vi "抽取1D数组(CTRL-REF).vi"(8 "error in (no error)":errorcluster caption="错误输入（无错误）", 10 "n":i32, 11 "输入数组":refnum<vi>[](array[refnum])) -> (0 "error out":errorcluster caption="错误输出", 3 "输出数组":refnum<vi>[][](array[refnum]))   [LabVIEW 2012]
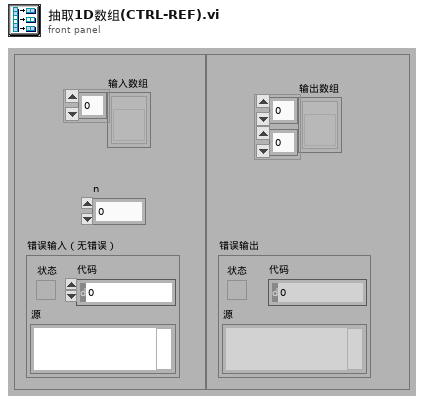
[diagram p1: front panel]
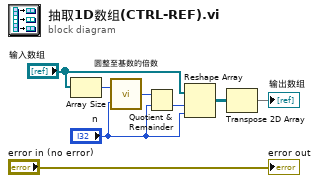
[diagram p0: block diagram]
diagram:
  n1 = Array Size(array="输入数组") -> (size(s)=w7:i32)
  n2 = call "圆整至基数的倍数.vi"("base"="n", "input"=w7) -> ("output"=w3:i32)
  n3 = Quotient & Remainder(x=w3, y="n") -> (floor(x/y)=w1:i32)  [unwired: 1 out]
  n4 = Reshape Array("输入数组", w1, "n") -> (w6:refnum<vi>[][])
  n5 = Transpose 2D Array(2D array=w6) -> (transposed array=→"输出数组":refnum<vi>[][])
  "error out" <- "error in (no error)"
